vi "Periodic Tasks.vi"(8 "error in":errorcluster) -> ()   [LabVIEW 2018]
doc: "This VI runs in parallel to other tasks. It can contain as many user-defined periodic loops as you need. These can carry out PID or other sorts of timed response."
uses:
  Swerve Drive/Vision Data.ctl
  <vilib>/Rock Robotics/WPI/Utilities/WPI_GetSetVariantRefNum.vi
  <vilib>/Rock Robotics/Network Tables/NT Write Boolean.vi
  <vilib>/Rock Robotics/Network Tables/NT Read Number.vi
  Robot Global Data.vi
  <vilib>/Rock Robotics/Network Tables/NT Write Number.vi
panel:
  out "Switch Pressed":bool
  out "Distance":dbl
  out "FR":dbl
  out "FL":dbl
  out "BR":dbl
  out "BL":dbl
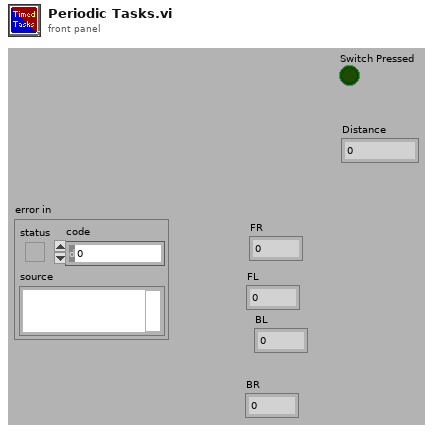
[diagram p1: front panel]
types:
  T1 = typedef "WPI_JoystickDevRef.ctl" = cluster{"Device":T2}
  T2 = typedef "WPI_JoystickDeviceEnum.ctl" = enum16{"USB 0", "USB 1", "USB 2", "USB 3", "USB 4", "USB 5"}
  T3 = typedef "WPI_SwitchDevRef.ctl" = cluster{"DevStatus":errorcluster, "DIO Channel":T4, "CntIndex":T5, "Normally Closed":bool}
  T4 = typedef "FPGA_DIOChannel.ctl" = enum8{"DIO 0", "DIO 1", "DIO 2", "DIO 3", "DIO 4", "DIO 5", "DIO 6", "DIO 7", "DIO 8", "DIO 9", "DIO MXP 0", "DIO MXP 1", "DIO MXP 2", "DIO MXP 3", "DIO MXP 4", "DIO MXP 5", "DIO MXP 6", "DIO MXP 7", "DIO MXP 8", "DIO MXP 9", "DIO MXP 10", "DIO MXP 11", "DIO MXP 12", "DIO MXP 13", "DIO MXP 14", "DIO MXP 15", "SPI Port CS1", "SPI Port CS2", "SPI Port CS3", "SPI Port MISO", "SPI Port MOSI", "Invalid"}
  T5 = typedef "FPGA_CounterCtrSystemIndex.ctl" = enum8{"Ctr 0", "Ctr 1", "Ctr 2", "Ctr 3", "Ctr 4", "Ctr 5", "Ctr 6", "Ctr 7", "Invalid"}
  T6 = typedef "WPI_CompressorDevRef.ctl" = cluster{"DevStatus":errorcluster, "Pneumatics Control Module":u8}
  T7 = typedef "Vision Data.ctl" = cluster{"xOffset":dbl, "yOffset":dbl, "area":dbl, "skewOffset":dbl, "hasTarget":dbl}
  T8 = cluster{"Yaw":dbl, "Roll":dbl, "Pitch":dbl, "Heading":dbl, "Fused Heading":dbl}
  T9 = typedef "WPI_AnalogChannelDevRef.ctl" = cluster{"DevStatus":errorcluster, "Analog Channel":T10}
  T10 = typedef "FPGA_AIChannel.ctl" = enum8{"AI 0", "AI 1", "AI 2", "AI 3", "AI MXP 0", "AI MXP 1", "AI MXP 2", "AI MXP 3", "Invalid"}
  T11 = typedef "WPI_EncoderDevRef.ctl" = cluster{"DevStatus":errorcluster, "EncoderIndex":T12, "CounterIndex":T5, "DistancePerCount":dbl, "Decoding Type":T13}
  T12 = typedef "FPGA_EncoderIdx.ctl" = enum8{"Enc 0", "Enc 1", "Enc 2", "Enc 3", "Enc 4", "Enc 5", "Enc 6", "Enc 7", "Invalid"}
  T13 = typedef "WPI_EncoderType.ctl" = enum16{"1x", "2x", "4x"}
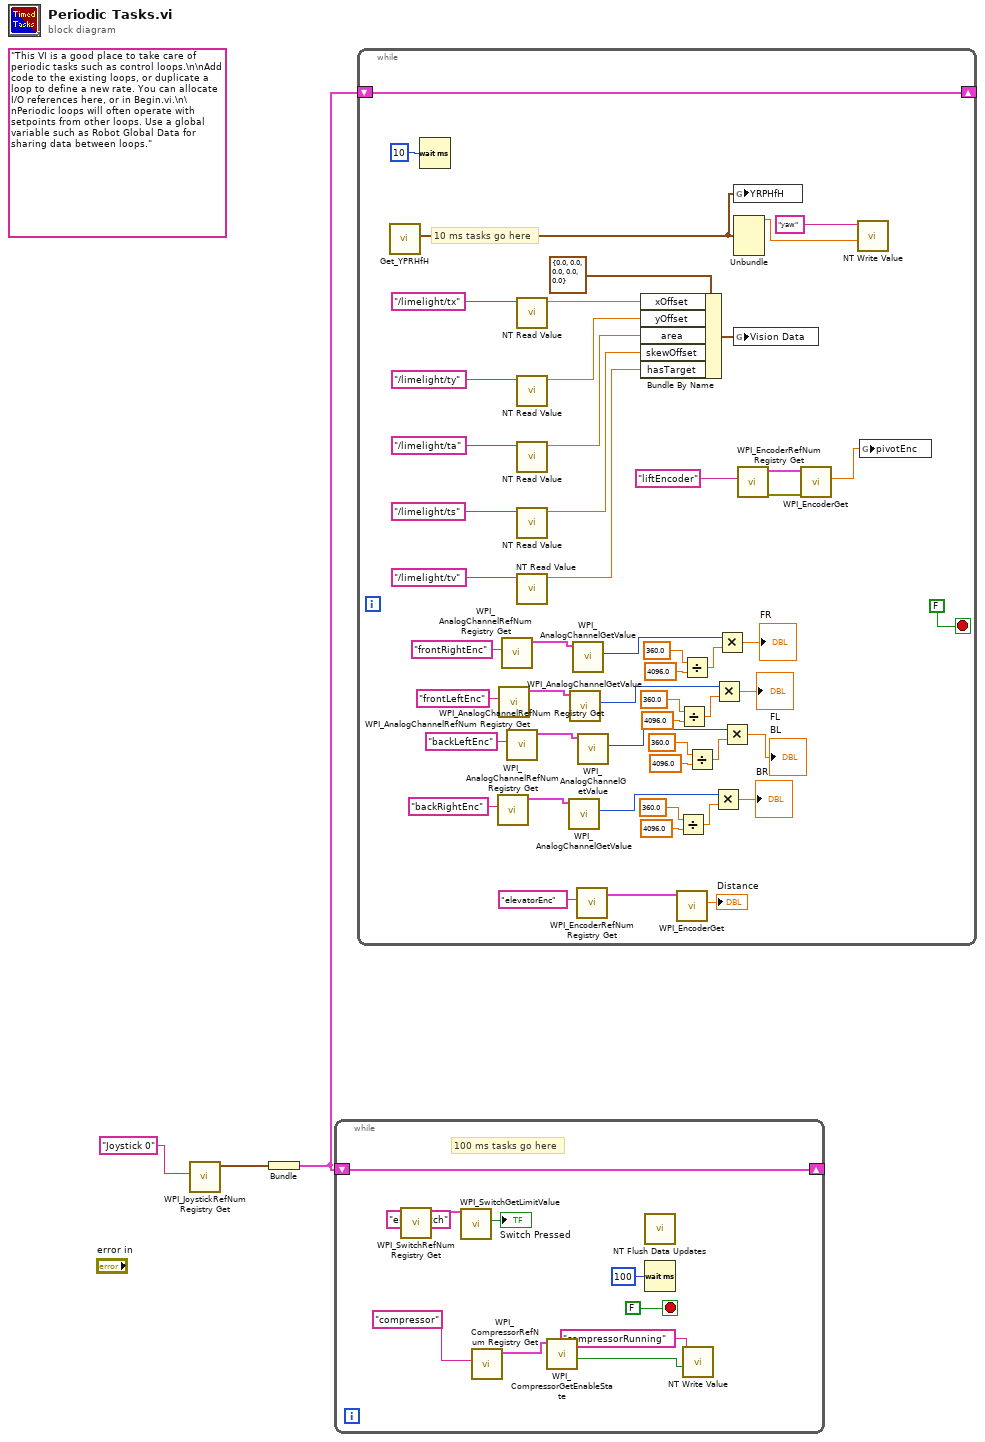
[diagram p0: block diagram]
diagram:
  (unwired) "This VI is a good place to take care of periodic tasks such as control loops.\n\nAdd code to the existing loops, or duplicate a loop to define a new rate. You can allocate I/O references here, or in Begin.vi.\n\nPeriodic loops will often operate with setpoints from other loops. Use a global variable such as Robot Global Data for sharing data between loops."
  n1 = call <vilib>:"WPI_JoystickRefNum Registry Get.vi"("refnum name"="Joystick 0") -> ("JoystickDevRef"=w2:T1)  [unwired: 1 in, 9 out]
  n2 = Bundle("JoystickDevRef"=w2) -> (w1:cluster{"JoystickDevRef":T1})  [unwired: 1 out]
  n3 = while {
    shift-right: [w11] -> _
    shift-left: w1 -> [w11]
    stop <- FALSE stop-if-true
    # "100 ms tasks go here"
    n4 = call <vilib>:"WPI_SwitchRefNum Registry Get.vi"("refnum name"="elevSwitch") -> ("SwitchDevRef"=w5:T3)  [unwired: 9 in, 1 out]
    n5 = call <vilib>:"WPI_SwitchGetLimitValue.vi"("SwitchDevRef"=w5) -> ("Switch Pressed"=→"Switch Pressed":bool)  [unwired: 8 in, 2 out]
    n6 = call <vilib>:"WPI_CompressorRefNum Registry Get.vi"("refnum name"="compressor") -> ("CompressorDevRef"=w9:T6)  [unwired: 9 in, 1 out]
    n7 = call <vilib>:"WPI_CompressorGetEnableState.vi"("CompressorDevRef"=w9) -> ("Compressor Running"=w8:bool)  [unwired: 7 in, 3 out]
    n8 = call <vilib>:"NT Flush Data Updates.vi"() -> ()  [unwired: 11 in, 1 out]
    n9 = Wait (ms)(milliseconds to wait=u32 100) -> ()  [unwired: 1 out]
    n10 = call-poly <vilib>:"NT Write Value.vi"("Boolean"=w8, "Name"="compressorRunning") -> ()  [unwired: 9 in, 1 out]
  }
  n11 = while {
    shift-right: [w49] -> _
    shift-left: w1 -> [w49]
    stop <- FALSE stop-if-true
    # "10 ms tasks go here"
    n12 = call <vilib>:"Get_YPRHfH.vi"() -> ("YRPHfH"=w52:T8)  [unwired: 11 in]
    n13 = Wait (ms)(milliseconds to wait=u32 10) -> ()  [unwired: 1 out]
    n14 = call <vilib>:"WPI_AnalogChannelRefNum Registry Get.vi"("refnum name"="backRightEnc") -> ("AIDeviceRef"=w35:T9)  [unwired: 9 in, 1 out]
    n15 = call <vilib>:"WPI_AnalogChannelRefNum Registry Get.vi"("refnum name"="frontLeftEnc") -> ("AIDeviceRef"=w34:T9)  [unwired: 9 in, 1 out]
    n16 = call <vilib>:"WPI_AnalogChannelRefNum Registry Get.vi"("refnum name"="frontRightEnc") -> ("AIDeviceRef"=w21:T9)  [unwired: 9 in, 1 out]
    n17 = call <vilib>:"WPI_AnalogChannelRefNum Registry Get.vi"("refnum name"="backLeftEnc") -> ("AIDeviceRef"=w48:T9)  [unwired: 9 in, 1 out]
    n18 = call-poly <vilib>:"NT Read Value.vi"("Name"="/limelight/tx") -> ("Numeric"=w62:dbl)  [unwired: 9 in, 1 out]
    n19 = call-poly <vilib>:"NT Read Value.vi"("Name"="/limelight/ty") -> ("Numeric"=w61:dbl)  [unwired: 9 in, 1 out]
    n20 = call-poly <vilib>:"NT Read Value.vi"("Name"="/limelight/ta") -> ("Numeric"=w60:dbl)  [unwired: 9 in, 1 out]
    n21 = call-poly <vilib>:"NT Read Value.vi"("Name"="/limelight/ts") -> ("Numeric"=w59:dbl)  [unwired: 9 in, 1 out]
    n22 = call-poly <vilib>:"NT Read Value.vi"("Name"="/limelight/tv") -> ("Numeric"=w58:dbl)  [unwired: 9 in, 1 out]
    n23 = call <vilib>:"WPI_AnalogChannelGetValue.vi"("AIDeviceRef"=w35) -> ("Value"=w39:i16)  [unwired: 8 in, 2 out]
    n24 = call <vilib>:"WPI_AnalogChannelGetValue.vi"("AIDeviceRef"=w34) -> ("Value"=w30:i16)  [unwired: 8 in, 2 out]
    n25 = call <vilib>:"WPI_AnalogChannelGetValue.vi"("AIDeviceRef"=w21) -> ("Value"=w25:i16)  [unwired: 8 in, 2 out]
    n26 = call <vilib>:"WPI_EncoderRefNum Registry Get.vi"("refnum name"="elevatorEnc") -> ("EncoderDevRef"=w19:T11)  [unwired: 9 in, 1 out]
    n27 = call <vilib>:"WPI_AnalogChannelGetValue.vi"("AIDeviceRef"=w48) -> ("Value"=w44:i16)  [unwired: 8 in, 2 out]
    n28 = Bundle By Name(cluster=T7 {"xOffset"=0.0, "yOffset"=0.0, "area"=0.0, "skewOffset"=0.0, "hasTarget"=0.0} ("Vision Data"), "xOffset"=w62, "yOffset"=w61, "area"=w60, "skewOffset"=w59, "hasTarget"=w58) -> (w63:T7)
    n29 = call <vilib>:"WPI_EncoderGet.vi"("EncoderDevRef"=w19) -> ("Distance"=→"Distance":dbl)  [unwired: 5 in, 5 out]
    n30 = Divide(x=360.0, y=4096.0) -> (x/y=w38:dbl)
    n31 = Divide(x=360.0, y=4096.0) -> (x/y=w31:dbl)
    n32 = Divide(x=360.0, y=4096.0) -> (x/y=w24:dbl)
    n33 = Divide(x=360.0, y=4096.0) -> (x/y=w45:dbl)
    n34 = Multiply(x=w39, y=w38) -> (x*y=→"BR":dbl)
    n35 = Multiply(x=w30, y=w31) -> (x*y=→"FL":dbl)
    n36 = Multiply(x=w25, y=w24) -> (x*y=→"FR":dbl)
    n37 = Multiply(x=w44, y=w45) -> (x*y=→"BL":dbl)
    n38 = global write "Robot Global Data.vi" "YRPHfH"(w52) -> ()
    n39 = Unbundle(w52) -> ("Yaw"=w51:dbl)  [unwired: 4 out]
    n40 = global write "Robot Global Data.vi" "Vision Data"(w63) -> ()
    n41 = call <vilib>:"WPI_EncoderRefNum Registry Get.vi"("refnum name"="liftEncoder") -> ("error out"=w15:errorcluster, "EncoderDevRef"=w16:T11)  [unwired: 9 in]
    n42 = call <vilib>:"WPI_EncoderGet.vi"("error in (no error)"=w15, "EncoderDevRef"=w16) -> ("Distance"=w14:dbl)  [unwired: 4 in, 5 out]
    n43 = call-poly <vilib>:"NT Write Value.vi"("Numeric"=w51, "Name"="yaw") -> ()  [unwired: 9 in, 1 out]
    n44 = global write "Robot Global Data.vi" "pivotEnc"(w14) -> ()
  }
